vi "dist and curvature.vi"(11 "Path":dbl[][](array[numeric])) -> (2 "Curvatures":dbl[](array[numeric]), 3 "Distances":dbl[](array[numeric]))   [LabVIEW 2018]
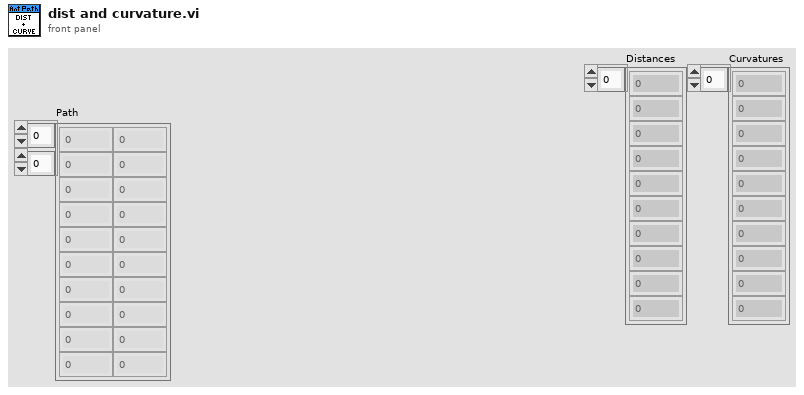
[diagram p1: front panel]
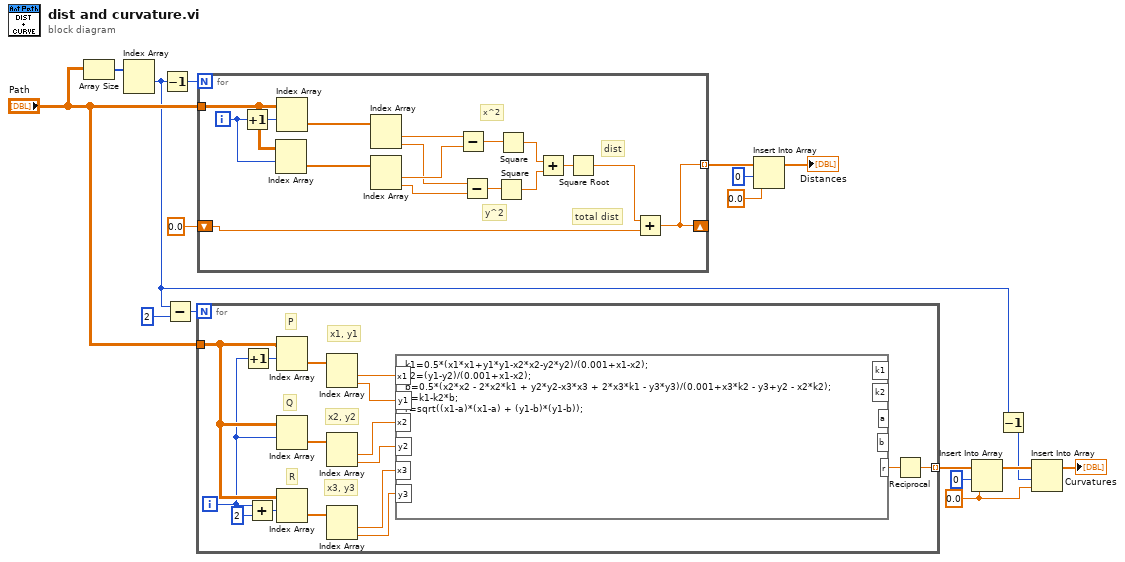
[diagram p0: block diagram]
diagram:
  w2 = 0.0 ("new element/subarray")
  n1 = Array Size(array="Path") -> (size(s)=w17:i32[])
  n2 = Index Array(array=w17) -> (element #1=w3:i32)  [unwired: 2 in, 1 out]
  n3 = Decrement(x=w3) -> (x-1=w16:i32)
  n4 = Subtract(x=w3, y=2) -> (x-y=w9:i32)
  n5 = for {
    N: w9 -> [_]
    tunnel: "Path" -> [w33]
    tunnel: [w18] -> w7 mode=indexing
    i -> [w31]
    # "x3, y3"
    # "x2, y2"
    # "x1, y1"
    # "R"
    # "Q"
    # "P"
    n6 = Increment(x=w31) -> (x+1=w32:i32)
    n7 = Add(x=w31, y=2) -> (x+y=w30:i32)
    n8 = Index Array(array=w33, index (row)=w32) -> (element=w28:dbl[])  [unwired: 1 in]
    n9 = Index Array(array=w33, index (row)=w31) -> (element=w27:dbl[])  [unwired: 1 in]
    n10 = Index Array(array=w33, index (row)=w30) -> (element=w26:dbl[])  [unwired: 1 in]
    n11 = Index Array(array=w28) -> (element #1=w25:dbl, element #2=w20:dbl)  [unwired: 2 in]
    n12 = Index Array(array=w27) -> (element #1=w24:dbl, element #2=w19:dbl)  [unwired: 2 in]
    n13 = Index Array(array=w26) -> (element #1=w23:dbl, element #2=w22:dbl)  [unwired: 2 in]
    n14 = formula code="k1=0.5*(x1*x1+y1*y1-x2*x2-y2*y2)/(0.001+x1-x2);\nk2=(y1-y2)/(0.001+x1-x2);\nb=0.5*(x2*x2 - 2*x2*k1 + y2*y2-x3*x3 + 2*x3*k1 - y3*y3)/(0.001+x3*k2 - y3+y2 - x2*k2);\na=k1-k2*b;\nr=sqrt((x1-a)*(x1-a) + (y1-b)*(y1-b));"("x1"=w25, "y1"=w20, "x2"=w24, "y2"=w19, "x3"=w23, "y3"=w22) -> ("r"=w21:dbl)  [unwired: 4 out]
    n15 = Reciprocal(x=w21) -> (1/x=w18:dbl)
  }
  n16 = for {
    N: w16 -> [_]
    tunnel: "Path" -> [w49]
    shift-right: [w35] -> _
    shift-left: 0.0 -> [w37]
    tunnel: [w35] -> w14 mode=indexing
    i -> [w50]
    # "total dist"
    # "dist"
    # "y^2"
    # "x^2"
    n17 = Increment(x=w50) -> (x+1=w34:i32)
    n18 = Index Array(array=w49, index (row)=w50) -> (element=w47:dbl[])  [unwired: 1 in]
    n19 = Index Array(array=w49, index (row)=w34) -> (element=w48:dbl[])  [unwired: 1 in]
    n20 = Index Array(array=w48) -> (element #1=w46:dbl, element #2=w43:dbl)  [unwired: 2 in]
    n21 = Index Array(array=w47) -> (element #1=w45:dbl, element #2=w42:dbl)  [unwired: 2 in]
    n22 = Subtract(x=w46, y=w45) -> (x-y=w44:dbl)
    n23 = Subtract(x=w43, y=w42) -> (x-y=w41:dbl)
    n24 = Square(x=w41) -> (x^2=w39:dbl)
    n25 = Square(x=w44) -> (x^2=w40:dbl)
    n26 = Add(x=w40, y=w39) -> (x+y=w38:dbl)
    n27 = Square Root(x=w38) -> (sqrt(x)=w36:dbl)
    n28 = Add(x=w36, y=w37) -> (x+y=w35:dbl)
  }
  n29 = Insert Into Array(array=w14, index=0, new element=0.0 ("new element/subarray")) -> (→"Distances":dbl[])
  n30 = Insert Into Array(array=w7, index=0, new element=w2) -> (w5:dbl[])
  n31 = Decrement(x=w3) -> (x-1=w1:i32)
  n32 = Insert Into Array(array=w5, index=w1, new element=w2) -> (→"Curvatures":dbl[])
